vi "svfa_Scaled Time Domain Window (NxM) (Dual).vi"(0 "stimulus signals X [EUx]":waveform(dbl)[](array[waveform]), 5 "response signals Y [EUy]":waveform(dbl)[](array[waveform]), 7 "window":T1=1 items=["None"=0, "Hanning"=1, "Hamming"=2, "Blackman-Harris"=3, "Exact Blackman"=4, "Blackman"=5, "Flat Top"=6, "4 Term B-Harris "=7, "7 Term B-Harris"=8, "Low Sidelobe"=9, "Force - Exponential"=10, "Force"=64, "Exponential"=65, "Blackman Nuttall"=11, "Triangle"=30, "Bartlett-Hanning"=31, "Bohman"=32, "Parzen"=33, "Welch"=34, "Kaiser"=60, "Dolph-Chebyshev"=61, "Gaussian"=62], 9 "Force - Exponential window settings":cluster{"force [%]":dbl, "exp [%]":dbl}={"force [%]"=50.0, "exp [%]"=10.0} {"exp [%]" min=0.0 max=100.0 format="%.2f"; "force [%]" min=0.0 max=100.0 format="%.2f"}, 11 "error in (no error)":errorcluster) -> (4 "windowed stimulus signals X [EUx]":waveform(dbl)[](array[waveform]), 6 "windowed response signals Y [EUy]":waveform(dbl)[](array[waveform]), 8 "window":T1 items=["None"=0, "Hanning"=1, "Hamming"=2, "Blackman-Harris"=3, "Exact Blackman"=4, "Blackman"=5, "Flat Top"=6, "4 Term B-Harris "=7, "7 Term B-Harris"=8, "Low Sidelobe"=9, "Force - Exponential"=10, "Force"=64, "Exponential"=65, "Blackman Nuttall"=11, "Triangle"=30, "Bartlett-Hanning"=31, "Bohman"=32, "Parzen"=33, "Welch"=34, "Kaiser"=60, "Dolph-Chebyshev"=61, "Gaussian"=62], 10 "window size":i32, 15 "error out":errorcluster)   [LabVIEW 2017]
doc: "Applies the selected window to the time-domain signal. The VI scales the result so that when the power or amplitude spectrum of the windowed waveform is computed, all windows provide the same level within the accuracy constraints of the window."
uses:
  <vilib>/addons/_NISVFA/_Shared subVIs/Controls/svc_Window [Dual FFT].ctl
  <vilib>/addons/_NISVFA/_Shared subVIs/Windowing/svfa_Scaled Time Domain Window (1 Ch).vi
  <vilib>/addons/_NISVFA/_Shared subVIs/Windowing/svfa_Scaled Time Domain Window (Array).vi
  <vilib>/Analysis/4window.llb/Force Window.vi
  <vilib>/Analysis/4window.llb/Force Window (DBL).vi
  <vilib>/Analysis/4window.llb/Exponential Window.vi
  <vilib>/Analysis/4window.llb/Exponential Window (DBL).vi
  <vilib>/Utility/error.llb/Error Cluster From Error Code.vi
  <vilib>/Analysis/0measdsp.llb/Scaled Time Domain Window.vi
  <vilib>/Analysis/0measdsp.llb/Scaled Time Domain Window (DBL).vi
  <vilib>/addons/_NISVFA/_Spectrum Processing/subVIs/svfa_Spectrum Info Window to windowTd Type Def.vi
  <vilib>/addons/_NISVFA/_Shared subVIs/Common/svc_Window Parameters.vi
  <vilib>/addons/_NISVFA/_Shared subVIs/Common/svc_Get Window Info.vi
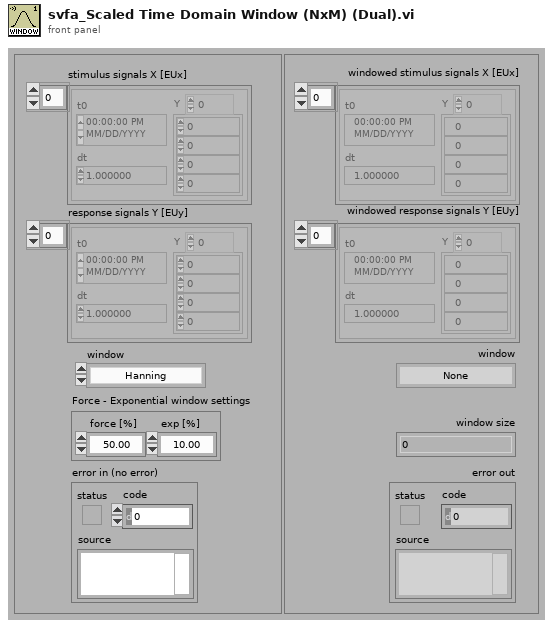
[diagram p1: front panel]
types:
  T1 = typedef "svc_Window [Dual FFT].ctl" = u32
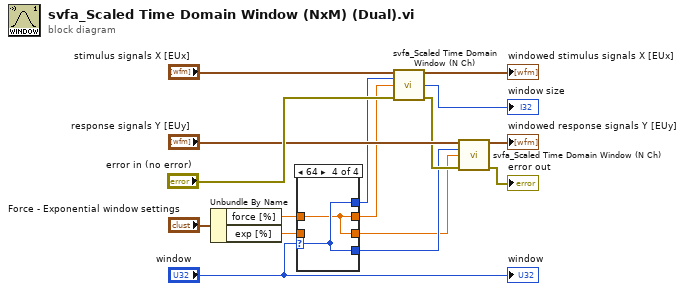
[diagram p0: block diagram]
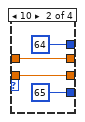
[diagram p3: hidden frame]
diagram:
  n1 = Unbundle By Name("Force - Exponential window settings") -> ("force [%]"=w8:dbl, "exp [%]"=w7:dbl)
  n2 = case shown="64" "window" {
    selector: "window" -> [w19 _ w25 w27]
    tunnel: [w19 u16 64 ("window") w25 w27] -> w5
    tunnel: [w19 u16 65 ("window") w25 w27] -> w4
    tunnel: [w18 w21 w24 w26] -> w3
    tunnel: w8 -> [w18 w21 _ w26]
    tunnel: [w17 w20 w24 w26] -> w2
    tunnel: w7 -> [w17 w20 w24 _]
    frame 0, Default {
    }
    frame 10 {
    }
    frame 65 {
    }
    frame 64 {
    }
  }
  n3 = call <vilib>:"svfa_Scaled Time Domain Window (N Ch).vi"("Scaled signal(s)"="stimulus signals X [EUx]", "window"=w5, "window parameter"=w3, "error in (no error)"="error in (no error)") -> ("Windowed Waveform(s)"=→"windowed stimulus signals X [EUx]":waveform(dbl)[], "window length"=→"window size":i32, "error out"=w10:errorcluster)  [unwired: 7 in, 2 out]
  n4 = call <vilib>:"svfa_Scaled Time Domain Window (N Ch).vi"("Scaled signal(s)"="response signals Y [EUy]", "window"=w4, "window parameter"=w2, "error in (no error)"=w10) -> ("Windowed Waveform(s)"=→"windowed response signals Y [EUy]":waveform(dbl)[], "error out"=→"error out":errorcluster)  [unwired: 7 in, 3 out]
  "window" <- "window"
